vi "Rotation Matrix.vi"(4 "Rotation Angle (rad)":dbl) -> (1 "Rotation Matrix":dbl[][](array[numeric]))   [LabVIEW 2013]
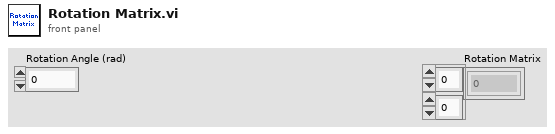
[diagram p1: front panel]
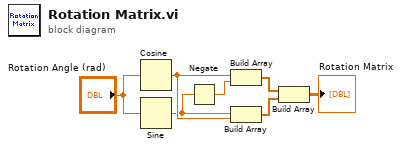
[diagram p0: block diagram]
diagram:
  n1 = Cosine(x="Rotation Angle (rad)") -> (cos(x)=w4:dbl)
  n2 = Sine(x="Rotation Angle (rad)") -> (sin(x)=w3:dbl)
  n3 = Negate(x=w3) -> (-x=w7:dbl)
  n4 = Build Array(w4, w7) -> (w6:dbl[])
  n5 = Build Array(w3, w4) -> (w5:dbl[])
  n6 = Build Array(w6, w5) -> (→"Rotation Matrix":dbl[][])
